vi "ComparadordeNumeros.vi"() -> ()   [LabVIEW 2022 SP3]
panel:
  in  "Stop Button":bool
  out "Boolean":bool
  in  "N 2":dbl
  in  "N1":dbl
  # "Comparación de dos números"
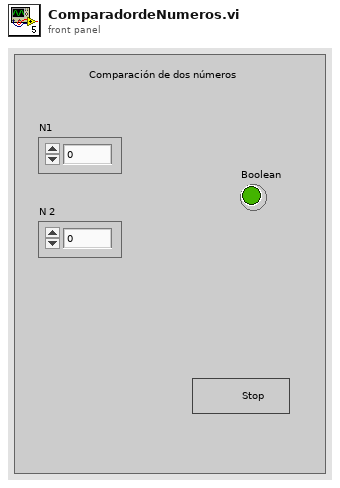
[diagram p1: front panel]
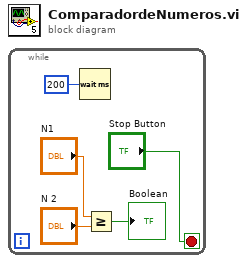
[diagram p0: block diagram]
diagram:
  n1 = while {
    stop <- "Stop Button" stop-if-true
    n2 = Wait (ms)(milliseconds to wait=u32 200 ("millisecond timer value")) -> ()  [unwired: 1 out]
    n3 = Greater Or Equal?(x="N1", y="N 2") -> (x >= y?=→"Boolean":bool)
  }
